vi "HTTPMethod1.vi"(7 "LabVIEW Web Service Request":refnum<class "Web Request.lvclass">) -> (0 "Fan2":bool, 1 "Fan1":bool, 2 "Hum":dbl, 3 "Temp":dbl)   [LabVIEW 2024]
uses:
  <vilib>/wsapi/Web Request.lvclass
  GlobalTemp1.vi
  GlobalFan1.vi
  GlobalFan2.vi
  GlobalHum1.vi
panel:
  # "Use the Web Service Request input terminal to call the VIs on the Web Services palette. Do not remove it from the connector pane unless you don't need access to the palette."
  # "Each additional control wired to the connector pane will be available as an input in the URL. To include an indicator in terminal-mode output (the default setting), it must also be wired to the connector pane."
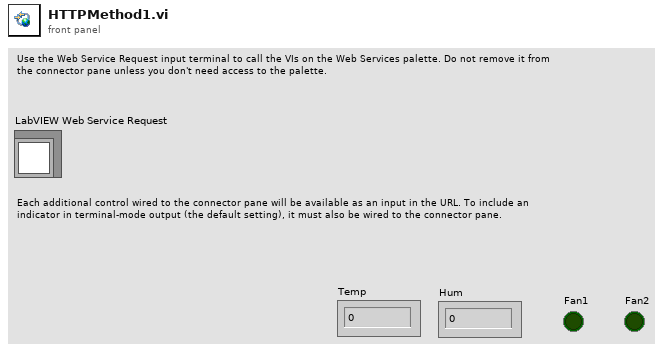
[diagram p1: front panel]
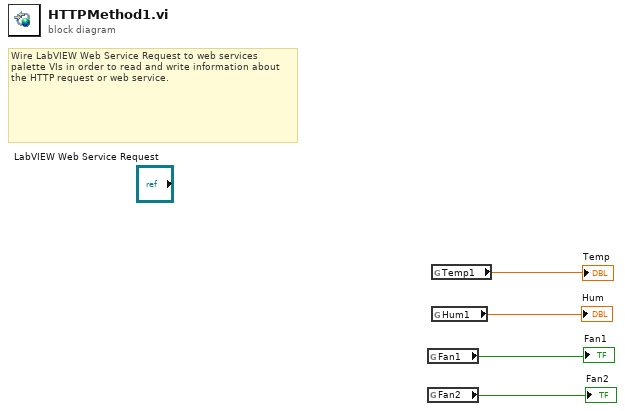
[diagram p0: block diagram]
diagram:
  # "Wire LabVIEW Web Service Request to web services palette VIs in order to read and write information about the HTTP request or web service."
  n1 = global read "GlobalFan1.vi" "Fan1"() -> (→"Fan1":bool)
  n2 = global read "GlobalFan2.vi" "Fan2"() -> (→"Fan2":bool)
  n3 = global read "GlobalTemp1.vi" "Temp1"() -> (→"Temp":dbl)
  n4 = global read "GlobalHum1.vi" "Hum1"() -> (→"Hum":dbl)
